vi "Labview_JFRM_while&for.vi"() -> ()   [LabVIEW 2020]
panel:
  out "Indice":i32[](array[numeric])
  out "Valor":dbl[](array[numeric])
  in  "stop":bool
  out "Random number generator":dbl
  in  "error constant":errorcluster
  out "Iteración":i32
  in  "Enable":bool
  # "Ciclo While"
  # "For Loop"
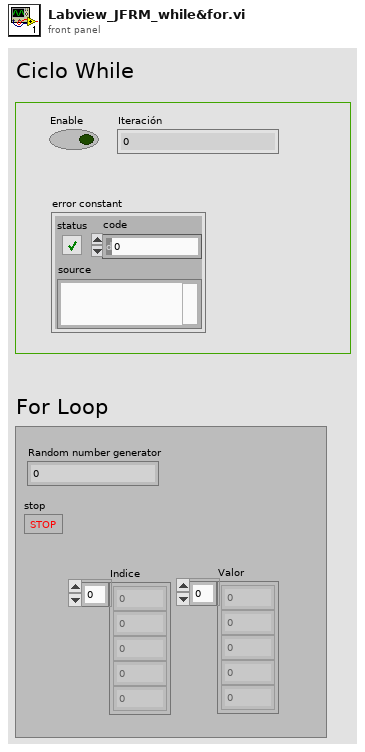
[diagram p1: front panel]
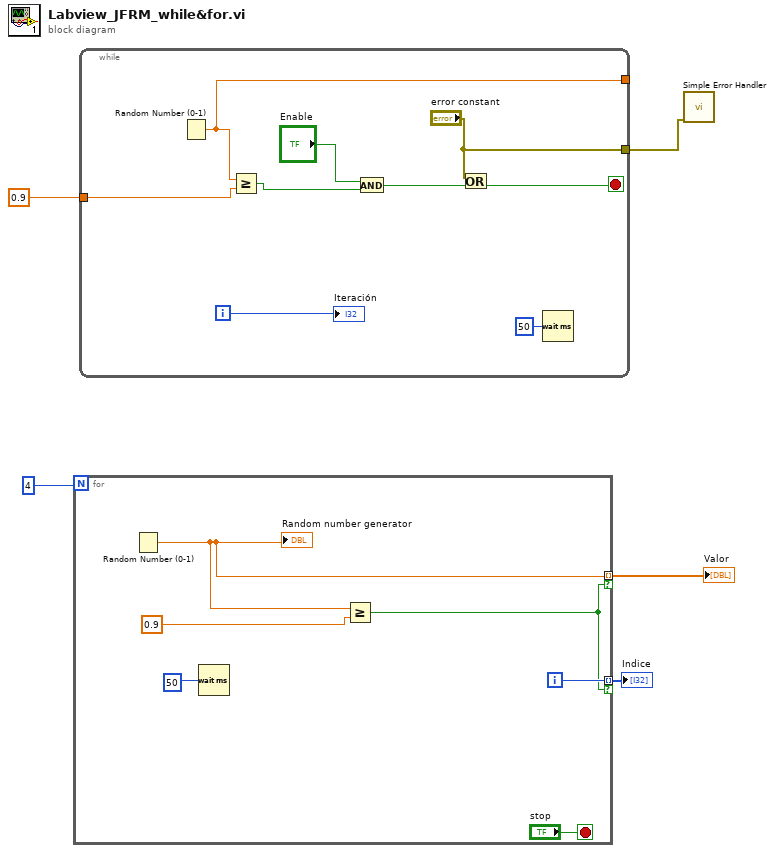
[diagram p0: block diagram]
diagram:
  n1 = for {
    N: 4 -> [_]
    tunnel: [w9] -> w3 mode=indexing if=w6
    tunnel: [w7] -> w2 mode=indexing if=w6
    i -> [w7]
    stop <- "stop" stop-if-true
    n2 = Random Number (0-1)() -> (number: 0 to 1=w9:dbl)
    "Random number generator" <- w9
    n3 = Wait (ms)(milliseconds to wait=u32 50 ("millisecond timer value")) -> ()  [unwired: 1 out]
    n4 = Greater Or Equal?(x=w9, y=0.9) -> (x >= y?=w6:bool)
  }
  "Valor" <- w3
  "Indice" <- w2
  n5 = while {
    tunnel: 0.9 -> [w20]
    tunnel: ["error constant"] -> w4
    tunnel: [w12] -> _
    i -> [w17]
    stop <- w15 stop-if-true
    n6 = Random Number (0-1)() -> (number: 0 to 1=w12:dbl)
    n7 = Greater Or Equal?(x=w12, y=w20) -> (x >= y?=w19:bool)
    n8 = And(x="Enable", y=w19) -> (x .and. y?=w14:bool)
    n9 = Or(x="error constant", y=w14) -> (x .or. y?=w15:bool)
    n10 = Wait (ms)(milliseconds to wait=u32 50) -> ()  [unwired: 1 out]
    "Iteración" <- w17
  }
  n11 = call <vilib>:"Simple Error Handler.vi"("error in (no error)"=w4) -> ()  [unwired: 4 in, 5 out]
